vi "Ctor.vi"(8 "error in (no error)":errorcluster, 11 "Team Field Panel in":refnum<class "Team Field Panel.lvclass">) -> (0 "error out":errorcluster, 3 "Team Field Panel out":refnum<class "Team Field Panel.lvclass">)   [LabVIEW 2020, in "SB App.lvlib" / "Team Field Panel.lvclass"]
uses:
  Team Field Panel.lvclass
  Team Map Update Data.ctl
  Team Field Panel.lvclass/Team Field Panel.ctl
  <vilib>/IlluminatedG/IG OOPanel/OOPanel/Panel/Panel.lvclass
  SB App.lvlib
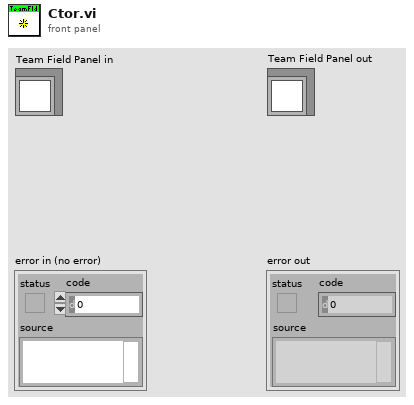
[diagram p1: front panel]
types:
  T1 = typedef "SB App.lvlib/Team Map Update Data.ctl" = cluster{"Team Map":i32[][]}
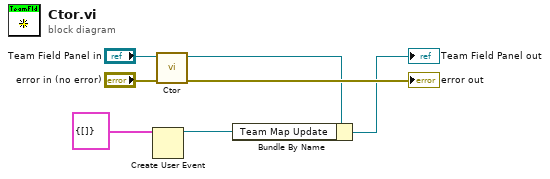
[diagram p0: block diagram]
diagram:
  n1 = Create User Event(user event datatype=T1 {"Team Map"=[]} ("Team Map Update Data")) -> (user event=w3:refnum<user-event>)  [unwired: 1 in, 1 out]
  n2 = call-parent "Ctor.vi"("error in (no error)"="error in (no error)", "Panel in"="Team Field Panel in") -> ("error out"=→"error out":errorcluster, "Panel out"=w2:refnum<class "Team Field Panel.lvclass">)  [unwired: 8 in]
  n3 = Bundle By Name(cluster=w2, "Team Map Update"=w3) -> (→"Team Field Panel out":refnum<class "Team Field Panel.lvclass">)
